vi "Elapsed Time.vi"(6 "Action":T1, 8 "Error In":errorcluster) -> (0 "Error Out":errorcluster, 1 "Elapsed Time [s]":dbl, 2 "Update Rate [1/s]":dbl)   [LabVIEW 2017]
uses:
  Controls/Global Variable Control.ctl
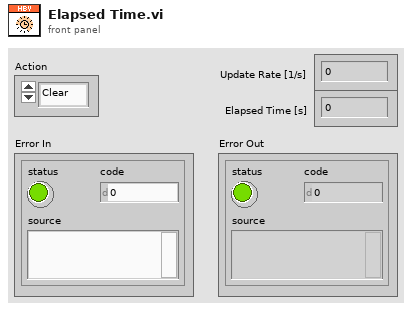
[diagram p1: front panel]
types:
  T1 = typedef "Global Variable Control.ctl" = enum16{"Clear", "Set", "Get"}
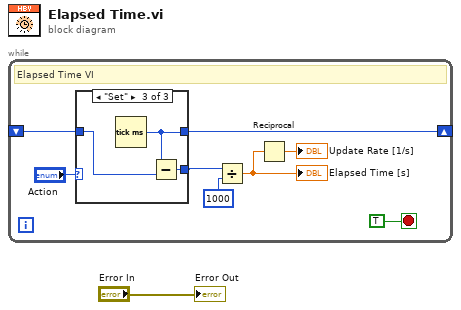
[diagram p0: block diagram]
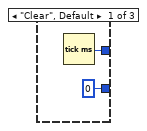
[diagram p2: hidden frame]
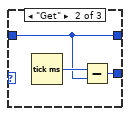
[diagram p3: hidden frame]
diagram:
  n1 = while {
    shift-right: [w7] -> _
    shift-left: _ -> [w6]
    stop <- TRUE stop-if-true
    # "Elapsed Time VI"
    n2 = case shown="\"Set\"" "Action" {
      tunnel: [w11 w13 w16] -> w7
      tunnel: w6 -> [_ w13 w17]
      tunnel: [u32 0 w12 w15] -> w5
      frame "Clear", Default {
        n3 = Tick Count (ms)() -> (millisecond timer value=w11:u32)
      }
      frame "Get" {
        n4 = Tick Count (ms)() -> (millisecond timer value=w14:u32)
        n5 = Subtract(x=w14, y=w13) -> (x-y=w12:u32)
      }
      frame "Set" {
        n6 = Tick Count (ms)() -> (millisecond timer value=w16:u32)
        n7 = Subtract(x=w16, y=w17) -> (x-y=w15:u32)
      }
    }
    n8 = Divide(x=w5, y=u32 1000) -> (x/y=w3:dbl)
    "Elapsed Time [s]" <- w3
    n9 = Reciprocal(x=w3) -> (1/x=→"Update Rate [1/s]":dbl)
  }
  "Error Out" <- "Error In"
